vi "Main.vi"(11 "Module Admin":refnum<class "Delacor_lib_QMH_Module Admin.lvclass">) -> ()   [LabVIEW 2018, in "DMM Module.lvlib"]
doc: "This template is based off of the Queued Message Handler design pattern and the Queued Message Handler project template that ships with LabVIEW.\n\nThe main difference is that the queue is private to this module and communication between modules is performed via Broadcast and Request events.\n\nRequest events are wrapped in public API methods and are handled in the Event Handling Loop (EHL) of this VI. Any module can register for Broadcast events sent by this module. The EHL generates messages based on user interface actions.\n\nThe Message Handling Loop (MHL) processes messages generated by the EHL, or by other messages. The messages are string values, so new messages can be added easily to the Message Cases case structure in the MHL. Each message cluster can also provide an optional value for Message Data, which is a variant that can be converted to whatever message-specific data is required.\n_____\nBased on DQMH Project Template 6.0.0.91."
uses:
  DMM Module.lvlib
  <vilib>/Delacor/Delacor QMH/Libraries/Module Admin_class/Delacor_lib_QMH_Module Admin.lvclass
  Module Data--cluster.ctl
  <vilib>/Delacor/Delacor QMH/Libraries/Message Queue_class/Delacor_lib_QMH_Message Queue.lvclass/Delacor_lib_QMH_Message Queue.ctl
  Stop Argument--cluster.ctl
  <vilib>/Delacor/Delacor QMH/Libraries/Module Admin_class/Delacor_lib_QMH_Module Admin.lvclass/Delacor_lib_QMH_Module Admin.ctl
  DMM init Argument--cluster.ctl
  config channel Argument--cluster.ctl
  Read DCV_DCI Argument--cluster.ctl
  Read DCV_DCI (Reply Payload)--cluster.ctl
  DMM Close Argument--cluster.ctl
  <vilib>/Utility/miscctls.llb/LVPointTypeDef.ctl
  <vilib>/Delacor/Delacor QMH/Libraries/Message Queue_class/Delacor_lib_QMH_Enqueue Message (Single).vi
  <vilib>/Delacor/Delacor QMH/Libraries/Module Admin_class/Delacor_lib_QMH_Get External Launch.vi
  <vilib>/Utility/error.llb/Error Cluster From Error Code.vi
  <vilib>/ErrorRing/Error Ring.xnode
  <vilib>/Delacor/Delacor QMH/Libraries/Message Queue_class/Delacor_lib_QMH_Message Queue.lvclass
  <instrlib>/DMM4/DMM4.lvlib
panel:
  in  "Sets to Display":u16(ring)=2 items=["1st Display", "2nd Display", "1st & 2nd Display"]
  out "DCI":dbl
  out "DCV":dbl
  in  "Read DCV, DCI Dual mode":bool
  in  "Config Channel":bool
  in  "Detector Rate":u8(ring) items=["SLOW", "MID", "FAST"]
  in  "DCI Range":dbl=0.5
  in  "DCV Range":dbl=200.0
  in  "Open&Init":bool caption="Open&init"
  in  "VISA resource name":refnum<visa-resource-name>
  out "error out":errorcluster
  out "Status":string
  in  "Simulate MHL Error":bool
  in  "Simulate EHL Error":bool
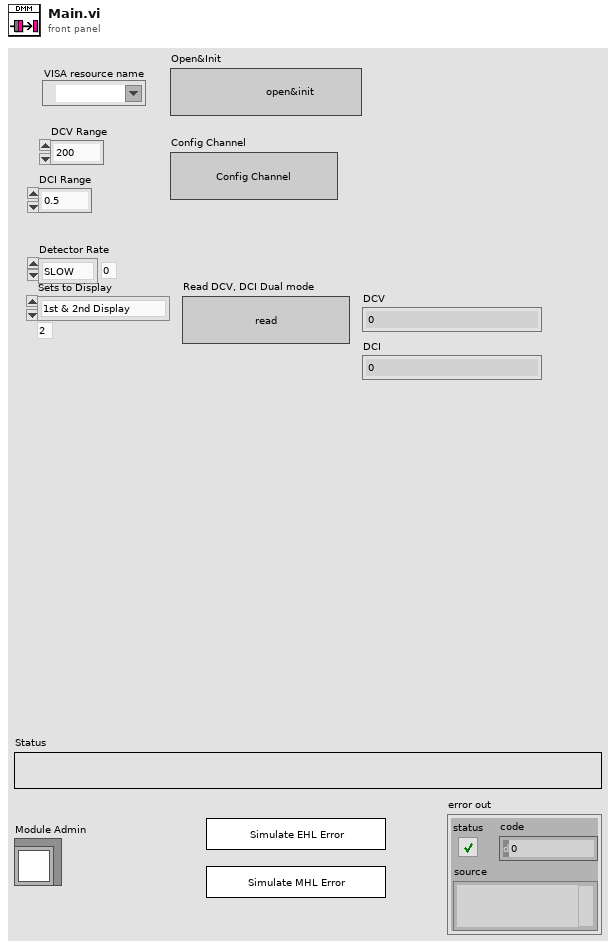
[diagram p1: front panel]
types:
  T1 = typedef "DMM Module.lvlib/Request Events--cluster.ctl" = cluster{"Stop Module":refnum<user-event>, "Do Something Else":refnum<user-event>, "Do Something Else and Wait for Reply":refnum<user-event>, "Show Panel":refnum<user-event>, "Hide Panel":refnum<user-event>, "Get Module Execution Status":refnum<user-event>, "Show Diagram":refnum<user-event>, "DMM init":refnum<user-event>, "config channel":refnum<user-event>, "Read DCV_DCI":refnum<user-event>, "DMM Close":refnum<user-event>}
  T2 = typedef "DMM Module.lvlib/Module Data--cluster.ctl" = cluster{"Status":string, "DMM  name":refnum<visa-resource-name>}
  T3 = typedef "LVPointTypeDef.ctl" = cluster{"Horizontal":i16, "Vertical":i16}
  T4 = enum32{"Invalid", "Standard", "Closed", "Hidden", "Minimized", "Maximized"}
  T5 = typedef "DMM Module.lvlib/DMM init Argument--cluster.ctl" = cluster{"VISA resource name":refnum<visa-resource-name>}
  T6 = typedef "DMM Module.lvlib/config channel Argument--cluster.ctl" = cluster{"Boolean":bool, "DCV range":dbl, "DCI range ":dbl, "Detector Rate":u8}
  T7 = typedef "DMM Module.lvlib/Read DCV_DCI (Reply Payload)--cluster.ctl" = cluster{"DCV":dbl, "DCI":dbl, "Read DCV_DCI_error":errorcluster}
  T8 = typedef "DMM Module.lvlib/Read DCV_DCI Argument--cluster.ctl" = cluster{"Wait Notifier":refnum<notifier>, "wait for reply":bool, "Sets to Display":u16}
  T9 = typedef "DMM Module.lvlib/DMM Close Argument--cluster.ctl" = cluster{"Boolean":bool}
  T10 = typedef "DMM Module.lvlib/Stop Argument--cluster.ctl" = cluster{"Origin":string, "Exit via Stop Module Req?":bool, "Wait for Module to stop?":bool}
  T11 = enum32{"invalid lock state", "Not Locked", "Locked (No Password)", "Password-protected"}
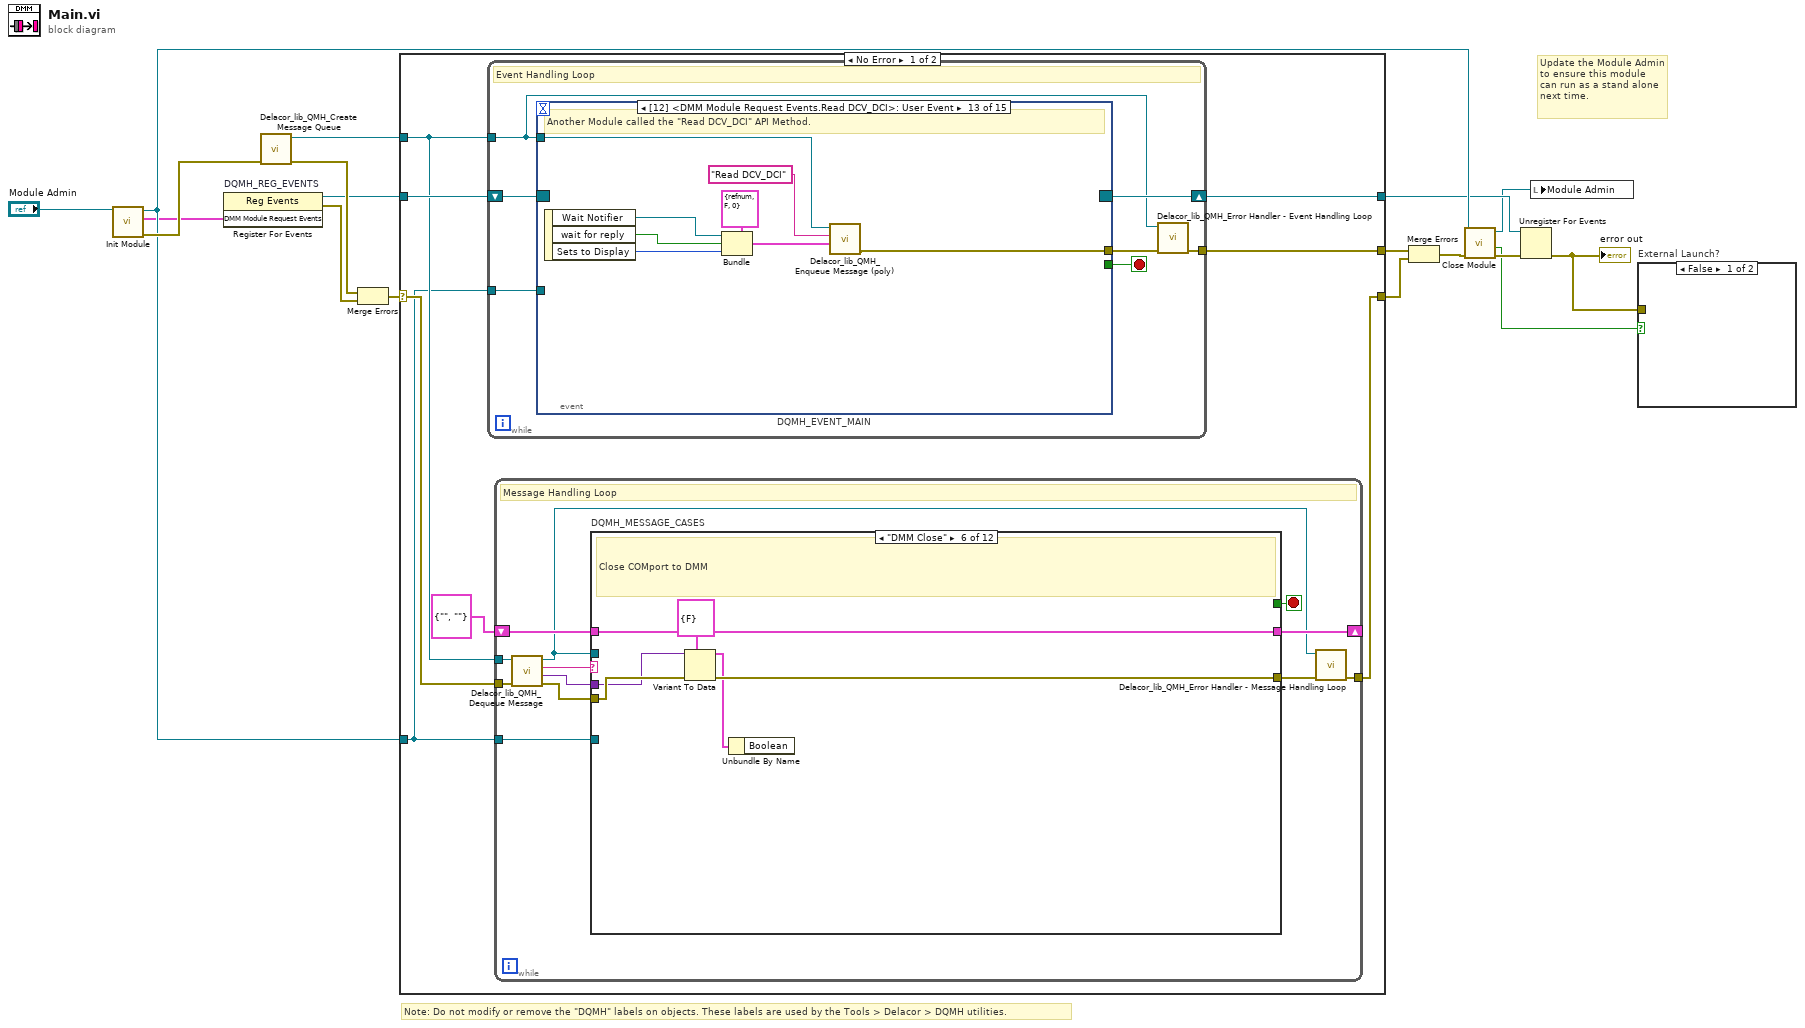
[diagram p0: block diagram]
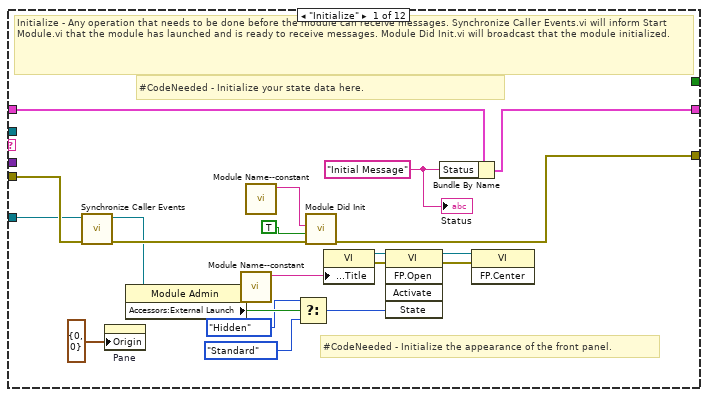
[diagram p2: hidden frame]
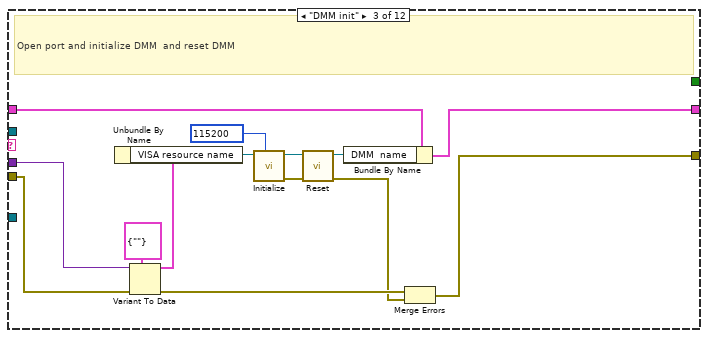
[diagram p4: hidden frame]
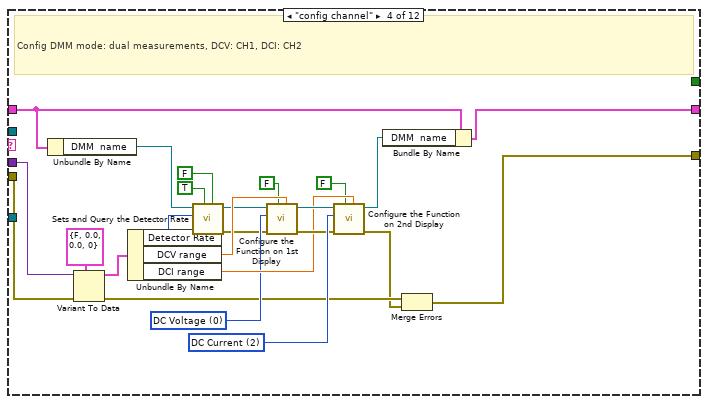
[diagram p5: hidden frame]
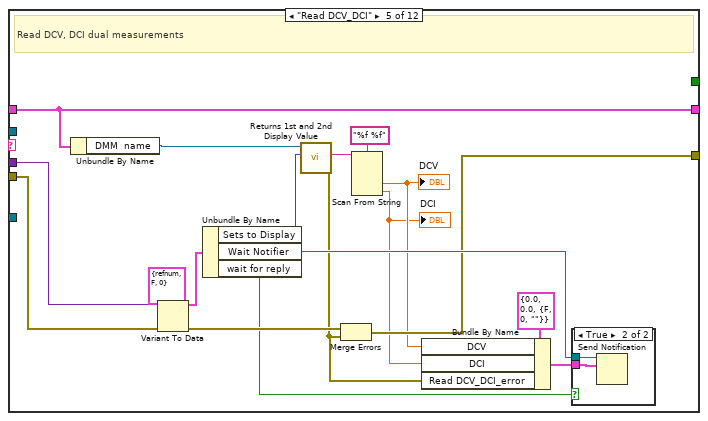
[diagram p6: hidden frame]
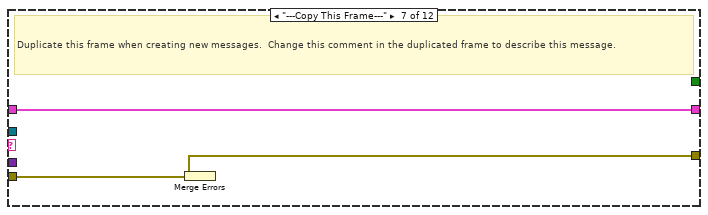
[diagram p8: hidden frame]
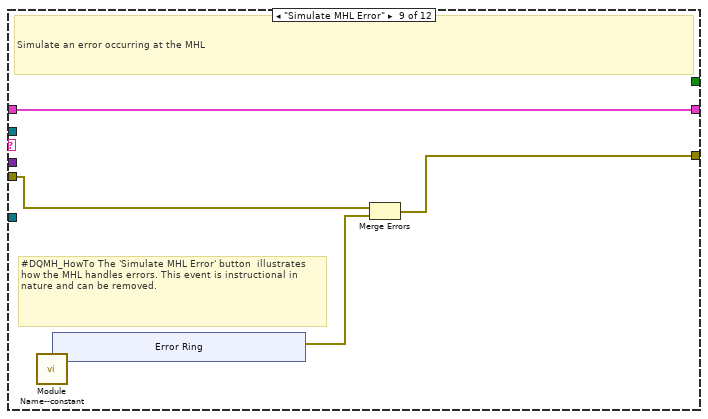
[diagram p10: hidden frame]
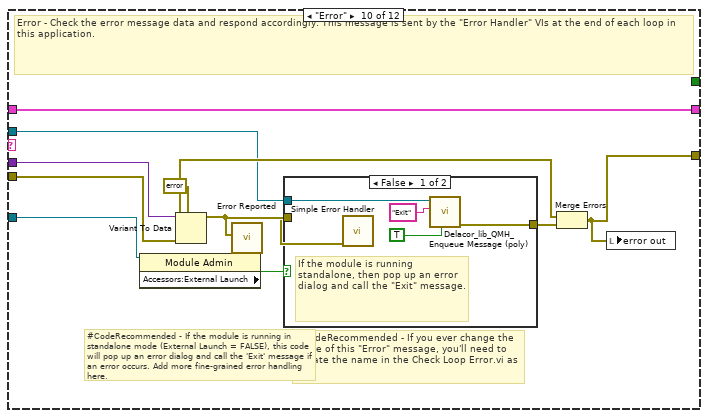
[diagram p11: hidden frame]
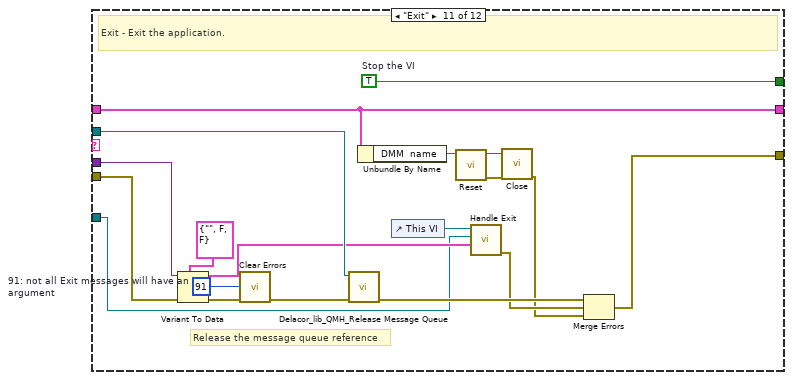
[diagram p13: hidden frame]
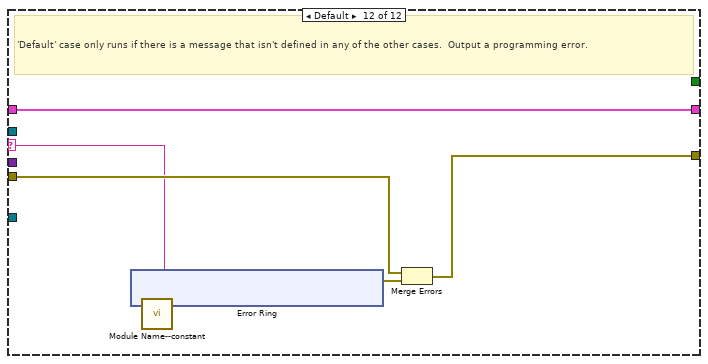
[diagram p14: hidden frame]
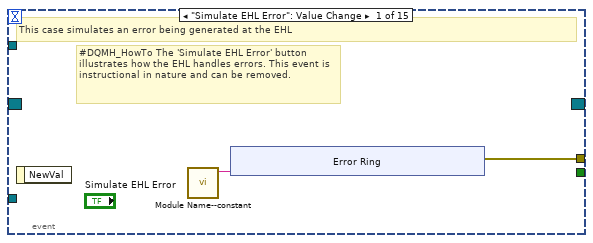
[diagram p15: hidden frame]
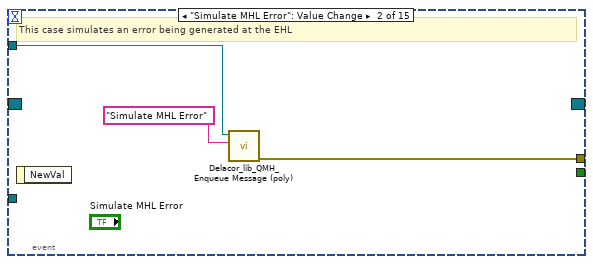
[diagram p16: hidden frame]
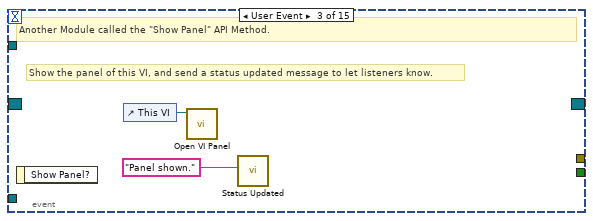
[diagram p17: hidden frame]
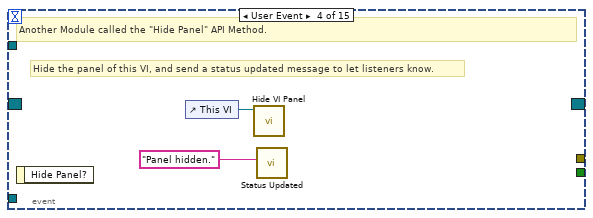
[diagram p18: hidden frame]
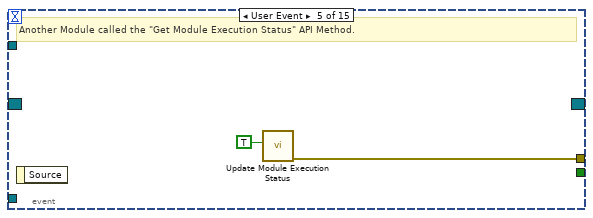
[diagram p19: hidden frame]
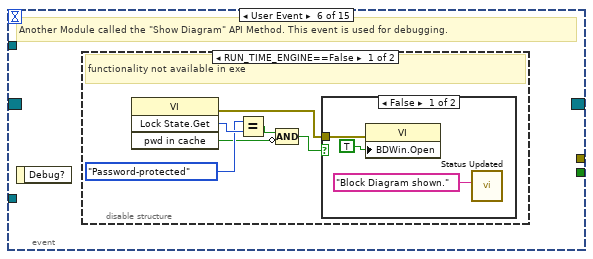
[diagram p20: hidden frame]
diagram:
  # "Note: Do not modify or remove the \"DQMH\" labels on objects. These labels are used by the Tools > Delacor > DQMH utilities."
  # "Update the Module Admin to ensure this module can run as a stand alone next time."
  n1 = call "Init Module.vi"("Singleton Module Admin in"="Module Admin") -> ("error out"=w16:errorcluster, "DMM Module Request Events"=w5:T1, "Singleton Module Admin out"=w8:refnum<class "Delacor_lib_QMH_Module Admin.lvclass">)  [unwired: 8 in]
  n2 = register-events "DQMH_REG_EVENTS"(w5) -> (reference out=w6:refnum<event-registration>, error out=w9:errorcluster)  [unwired: 2 in]
  n3 = call <vilib>:"Delacor_lib_QMH_Create Message Queue.vi"("error in"=w16) -> ("error out"=w11:errorcluster, "Message Queue"=w4:refnum<class "Delacor_lib_QMH_Message Queue.lvclass">)  [unwired: 9 in]
  n4 = Merge Errors(w11, w9) -> (w10:errorcluster)
  n5 = case shown="No Error" w10 {
    selector: w10 -> [w23 w297]
    tunnel: [w25 w296] -> w17
    tunnel: [w22 w302] -> w7
    tunnel: w6 -> [w20 w302]
    tunnel: w4 -> [w19 w295]
    tunnel: [w24 _] -> w14
    tunnel: w8 -> [w18 w298]
    frame No Error {
      n6 = while {
        tunnel: w19 -> [w190]
        shift-right: [w193] -> w22
        shift-left: w20 -> [w194]
        tunnel: [w195] -> w24
        tunnel: w18 -> [w191]
        stop <- w192 stop-if-true
        # "Event Handling Loop"
        n7 = event "DQMH_EVENT_MAIN" shown="[12] <DMM Module Request Events.Read DCV_DCI>: User Event" {
          selector: w194 -> [_ _ _ _ _ _ _ _ _ _ _ _ _ _ _]
          dyn-events: [_ _ _ _ _ _ _ _ _ _ _ _ _ _ _] -> w193
          timeout: _ -> [_ _ _ _ _ _ _ _ _ _ _ _ _ _ _]
          tunnel: [_ _ _ _ _ _ TRUE ("Discard?") _ _ _ _ _ _ _ _] -> w192
          tunnel: w190 -> [_ w207 _ _ _ _ w224 w238 w251 w256 w266 w269 w282 w288 w294]
          tunnel: [w198 w208 _ _ w214 _ w234 w240 w246 w252 w261 w267 w276 w283 w289] -> w196
          tunnel: w191 -> [_ _ _ _ _ _ _ w237 _ _ _ _ _ _ _]
          event "Simulate EHL Error": Value Change {
            # "#DQMH_HowTo The 'Simulate EHL Error' button  illustrates how the EHL handles errors. This event is instructional in nature and can be removed."
            # "This case simulates an error being generated at the EHL"
            n8 = event-data() -> ()  [unwired: 1 in, 1 out]
            n9 = call "Module Name--constant.vi"() -> ("Module Name"=w197:string)  [unwired: 11 in]
            n10 = xnode "Error Ring"("parameter 0"=w197) -> ("error out"=w198:errorcluster)
          }
          event "Simulate MHL Error": Value Change {
            # "This case simulates an error being generated at the EHL"
            n11 = event-data() -> ()  [unwired: 1 in, 1 out]
            n12 = call-poly <vilib>:"Delacor_lib_QMH_Enqueue Message (poly).vi"("Message"="Simulate MHL Error", "Message Queue in"=w207) -> ("error out"=w208:errorcluster)  [unwired: 8 in, 1 out]
          }
          event User Event {
            # "Show the panel of this VI, and send a status updated message to let listeners know."
            # "Another Module called the \"Show Panel\" API Method."
            n13 = event-data() -> ()  [unwired: 1 in, 1 out]
            n14 = control-ref of="This VI"() -> (w210:refnum<vi>)
            n15 = call "Open VI Panel.vi"("VI"=w210) -> ()  [unwired: 10 in, 1 out]
            n16 = call "Status Updated.vi"("Status"="Panel shown." ("format string")) -> ()  [unwired: 10 in, 1 out]
          }
          event User Event {
            # "Hide the panel of this VI, and send a status updated message to let listeners know."
            # "Another Module called the \"Hide Panel\" API Method."
            n17 = event-data() -> ()  [unwired: 1 in, 1 out]
            n18 = control-ref of="This VI"() -> (w212:refnum<vi>)
            n19 = call "Hide VI Panel.vi"("VI"=w212) -> ()  [unwired: 10 in, 1 out]
            n20 = call "Status Updated.vi"("Status"="Panel hidden." ("format string")) -> ()  [unwired: 10 in, 1 out]
          }
          event User Event {
            # "Another Module called the \"Get Module Execution Status\" API Method."
            n21 = event-data() -> ()  [unwired: 1 in, 1 out]
            n22 = call "Update Module Execution Status.vi"("Running?"=TRUE) -> ("error out"=w214:errorcluster)  [unwired: 10 in]
          }
          event User Event {
            # "Another Module called the \"Show Diagram\" API Method. This event is used for debugging."
            n23 = event-data() -> ()  [unwired: 1 in, 1 out]
            n24 = disable-structure shown="RUN_TIME_ENGINE==False" {
              frame condition #0 (active) {
                # "functionality not available in exe"
                n25 = invoke class="VI" method="Lock State.Get"() -> (error out=w220:errorcluster, "Get Lock State"=w219:T11, "pwd in cache"=w216:bool)  [unwired: 4 in, 1 out]
                n26 = Equal?(x=T11."Password-protected", y=w219) -> (x = y?=w217:bool)
                n27 = Compound Arithmetic op=AND(w217, invert w216) -> (w215:bool)
                n28 = case shown="False" w215 {
                  tunnel: w220 -> [w223 _]
                  frame False {
                    n29 = property class="VI"(error in=w223, "BDWin.Open"=TRUE ("Block Diagram Window:Open")) -> ()  [unwired: 1 in, 2 out]
                    n30 = call "Status Updated.vi"("Status"="Block Diagram shown." ("format string")) -> ()  [unwired: 10 in, 1 out]
                  }
                  frame True {
                    # "Password-protected VI, and the password is not in the cache. Do not show the diagram."
                  }
                }
              }
              frame condition #1 {
              }
            }
          }
          event User Event {
            # "The Stop Module Event can get fired from the Exit message in the MHL. The queue gets destroyed in that case. If the queue no longer exists, the Enqueue Exit as a priority message will return error 1. It is safe to ignore, because the module is already exiting."
            # "Another Module called the \"Stop Module\" API Method  or the Message Handling Loop below."
            n31 = event-data() -> ("Origin"=w231:string, "Exit via Stop Module Req?"=w227:bool, "Wait for Module to stop?"=w226:bool)  [unwired: 1 in]
            n32 = local write "Status"(w231) -> ()
            n33 = Bundle By Name(cluster=T10 {"Origin"="", "Exit via Stop Module Req?"=FALSE, "Wait for Module to stop?"=FALSE} ("Stop Argument"), "Exit via Stop Module Req?"=w227, "Wait for Module to stop?"=w226) -> (w225:T10)
            n34 = call-poly <vilib>:"Delacor_lib_QMH_Enqueue Message (poly).vi"("Priority Message? (F)"=TRUE, "Message Data"=w225, "Message"="Exit", "Message Queue in"=w224) -> ("error out"=w235:errorcluster)  [unwired: 6 in, 1 out]
            n35 = call <vilib>:"Clear Errors.vi"("error in (no error)"=w235, "specific error code to clear (0: all)"=1) -> ("error out"=w234:errorcluster)  [unwired: 4 in, 1 out]
          }
          event Panel Close? {
            w239 = TRUE  # Discard the event, the MHL is responsible for closing and stopping this VI.
            # "Hide the panel or send the 'Exit' message if the user clicks the 'X' on the module main VI panel."
            n36 = event-data() -> ()  [unwired: 1 in, 1 out]
            n37 = property class="Module Admin"(reference=w237) -> ("Accessors:External Launch"=w236:bool)  [unwired: 1 in, 2 out]
            n38 = case shown="False" w236 {
              tunnel: w238 -> [_ w244]
              tunnel: [_ w245] -> w240
              frame True {
                # "If externally launched, clicking the 'X' hides the panel, but doesn't close it."
                n39 = control-ref of="This VI"() -> (w241:refnum<vi>)
                n40 = call "Hide VI Panel.vi"("VI"=w241) -> ()  [unwired: 10 in, 1 out]
              }
              frame False {
                # "If run as a stand-alone VI, clicking the panel 'X' stops the VI."
                n41 = call-poly <vilib>:"Delacor_lib_QMH_Enqueue Message (poly).vi"("Priority Message? (F)"=TRUE, "Message"="Exit", "Message Queue in"=w244) -> ("error out"=w245:errorcluster)  [unwired: 7 in, 1 out]
              }
            }
            n42 = event-data("Discard?"=w239) -> ()  [unwired: 1 in, 1 out]
          }
          event User Event {
            # "Another Module called the \"DMM init\" API Method."
            n43 = event-data() -> ("VISA resource name"=w247:refnum<visa-resource-name>)  [unwired: 1 in]
            n44 = Bundle(cluster=T5 {"VISA resource name"=""} ("DMM init Argument"), "VISA resource name"=w247) -> (w248:T5)
            n45 = call-poly <vilib>:"Delacor_lib_QMH_Enqueue Message (poly).vi"("Message Data"=w248, "Message"="DMM init", "Message Queue in"=w251) -> ("error out"=w246:errorcluster)  [unwired: 7 in, 1 out]
          }
          event "Open&Init": Value Change {
            n46 = event-data() -> ()  [unwired: 1 in, 1 out]
            n47 = Bundle By Name(cluster=T5 {"VISA resource name"=""} ("DMM init Argument"), "VISA resource name"="VISA resource name") -> (w253:T5)
            n48 = call-poly <vilib>:"Delacor_lib_QMH_Enqueue Message (poly).vi"("Message Data"=w253, "Message"="DMM init", "Message Queue in"=w256) -> ("error out"=w252:errorcluster)  [unwired: 7 in, 1 out]
          }
          event User Event {
            # "Another Module called the \"config channel\" API Method."
            n49 = event-data() -> ("Boolean"=w262:bool, "DCV range"=w260:dbl, "DCI range"=w259:dbl, "Detector Rate"=w258:u8)  [unwired: 1 in]
            n50 = Bundle(cluster=T6 {"Boolean"=FALSE, "DCV range"=0.0, "DCI range "=0.0, "Detector Rate"=0} ("config channel Argument"), "Boolean"=w262, "DCV range"=w260, "DCI range"=w259, "Detector Rate"=w258) -> (w263:T6)
            n51 = call-poly <vilib>:"Delacor_lib_QMH_Enqueue Message (poly).vi"("Message Data"=w263, "Message"="config channel", "Message Queue in"=w266) -> ("error out"=w261:errorcluster)  [unwired: 7 in, 1 out]
          }
          event "Config Channel": Value Change {
            n52 = event-data() -> ()  [unwired: 1 in, 1 out]
            n53 = Bundle By Name(cluster=T6 {"Boolean"=FALSE, "DCV range"=0.0, "DCI range "=0.0, "Detector Rate"=0} ("config channel Argument"), "DCV range"="DCV Range", "DCI range"="DCI Range", "Detector Rate"="Detector Rate") -> (w268:T6)
            n54 = call-poly <vilib>:"Delacor_lib_QMH_Enqueue Message (poly).vi"("Message Data"=w268, "Message"="config channel", "Message Queue in"=w269) -> ("error out"=w267:errorcluster)  [unwired: 7 in, 1 out]
          }
          event User Event {
            # "Another Module called the \"Read DCV_DCI\" API Method."
            n55 = event-data() -> ("Wait Notifier"=w278:refnum<notifier>, "wait for reply"=w277:bool, "Sets to Display"=w275:u16)  [unwired: 1 in]
            n56 = Bundle(cluster=T8 {"Wait Notifier"=refnum, "wait for reply"=FALSE, "Sets to Display"=0} ("Read DCV_DCI Argument"), "Wait Notifier"=w278, "wait for reply"=w277, "Sets to Display"=w275) -> (w279:T8)
            n57 = call-poly <vilib>:"Delacor_lib_QMH_Enqueue Message (poly).vi"("Message Data"=w279, "Message"="Read DCV_DCI", "Message Queue in"=w282) -> ("error out"=w276:errorcluster)  [unwired: 7 in, 1 out]
          }
          event "Read DCV, DCI Dual mode": Value Change {
            n58 = event-data() -> ()  [unwired: 1 in, 1 out]
            n59 = Bundle By Name(cluster=T8 {"Wait Notifier"=refnum, "wait for reply"=FALSE, "Sets to Display"=0} ("Read DCV_DCI Argument"), "Sets to Display"="Sets to Display") -> (w284:T8)
            n60 = call-poly <vilib>:"Delacor_lib_QMH_Enqueue Message (poly).vi"("Message Data"=w284, "Message"="Read DCV_DCI", "Message Queue in"=w288) -> ("error out"=w283:errorcluster)  [unwired: 7 in, 1 out]
          }
          event User Event {
            # "Another Module called the \"DMM Close\" API Method."
            n61 = event-data() -> ("Boolean"=w290:bool)  [unwired: 1 in]
            n62 = Bundle(cluster=T9 {"Boolean"=FALSE} ("DMM Close Argument"), "Boolean"=w290) -> (w291:T9)
            n63 = call-poly <vilib>:"Delacor_lib_QMH_Enqueue Message (poly).vi"("Message Data"=w291, "Message"="DMM Close", "Message Queue in"=w294) -> ("error out"=w289:errorcluster)  [unwired: 7 in, 1 out]
          }
        }
        n64 = call-dynamic "Delacor_lib_QMH_Error Handler - Event Handling Loop.vi"("error in"=w196, "Message Queue in"=w190) -> ("dup error in"=w195:errorcluster)  [unwired: 8 in, 1 out]
      }
      n65 = while {
        tunnel: w19 -> [w28]
        shift-right: [w32] -> _
        shift-left: T2 {"Status"="", "DMM  name"=""} ("Data Cluster") -> [w33]
        tunnel: w23 -> [w36]
        tunnel: [w34] -> w25
        tunnel: w18 -> [w26]
        stop <- w31 stop-if-true
        # "Message Handling Loop"
        n66 = call-dynamic "Delacor_lib_QMH_Dequeue Message.vi"("error in"=w36, "Message Queue in"=w28) -> ("error out"=w35:errorcluster, "Message Data"=w29:variant, "Message"=w30:string, "Message Queue out"=w27:refnum<class "Delacor_lib_QMH_Message Queue.lvclass">)  [unwired: 6 in]
        n67 = case "DQMH_MESSAGE_CASES" shown="\"DMM Close\"" w30 {
          selector: w30 -> [_ _ _ _ _ _ _ _ _ _ _ w177]
          tunnel: w27 -> [_ _ _ _ _ _ _ _ _ w144 w169 _]
          tunnel: w35 -> [w55 w59 w73 w97 w115 w123 w126 w128 w133 w150 w175 w179]
          tunnel: [w53 w59 w62 w88 w106 w121 w125 w128 w132 w147 w172 w180] -> w37
          tunnel: w33 -> [w44 w58 w66 w89 w105 w122 w124 w127 w130 w146 w161 w178]
          tunnel: [w43 w58 w67 w90 w105 w122 w124 w127 w130 w146 w161 w178] -> w32
          tunnel: [_ _ _ _ _ _ _ _ _ _ w168 _] -> w31
          tunnel: w29 -> [_ _ w72 w96 w113 w120 _ _ _ w145 w167 _]
          tunnel: w26 -> [w45 _ _ _ _ _ _ _ _ w143 w162 _]
          frame "Initialize" {
            w39 = "Initial Message" ("Initial Message")
            # "#CodeNeeded - Initialize the appearance of the front panel."
            # "#CodeNeeded - Initialize your state data here."
            # "Initialize - Any operation that needs to be done before the module can receive messages. Synchronize Caller Events.vi will inform Start Module.vi that the module has launched and is ready to receive messages. Module Did Init.vi will broadcast that the module initialized."
            n68 = call "Synchronize Caller Events.vi"("error in (no error)"=w55, "Singleton Module Admin in"=w45) -> ("error out"=w54:errorcluster, "Singleton Module Admin out"=w40:refnum<class "Delacor_lib_QMH_Module Admin.lvclass">)  [unwired: 8 in]
            n69 = property on="Pane" class="Pane"("Origin"=T3 {"Horizontal"=0, "Vertical"=0}) -> ()  [unwired: 2 in, 2 out]
            n70 = property class="Module Admin"(reference=w40) -> ("Accessors:External Launch"=w49:bool)  [unwired: 1 in, 2 out]
            n71 = call "Module Name--constant.vi"() -> ("Module Name"=w52:string)  [unwired: 11 in]
            n72 = call "Module Name--constant.vi"() -> ("Module Name"=w41:string)  [unwired: 11 in]
            n73 = Select(t=T4."Hidden" ("State"), s=w49, f=T4."Standard" ("State")) -> (s? t:f=w46:T4)
            n74 = call "Module Did Init.vi"("error in (no error)"=w54, "Initialized?"=TRUE, "Origin"=w41) -> ("error out"=w53:errorcluster)  [unwired: 8 in]
            n75 = property class="VI"("Front Panel.Title"=w52) -> (reference out=w51:refnum<vi>, error out=w57:errorcluster)  [unwired: 2 in]
            n76 = invoke class="VI" method="FP.Open"(reference=w51, error in=w57, "State"=w46) -> (reference out=w50:refnum<vi>, error out=w56:errorcluster)  [unwired: 2 in, 3 out]
            n77 = Bundle By Name(cluster=w44, "Status"=w39) -> (w43:T2)
            n78 = invoke class="VI" method="FP.Center"(reference=w50, error in=w56) -> ()  [unwired: 1 in, 3 out]
            "Status" <- w39
          }
          frame "---Module Specific---" {
            # "Separator -- The following cases handle messages specific to this Module."
          }
          frame "DMM init" {
            w68 = u32 115200 items=["9600"=9600, "19200"=19200, "38400"=38400, "57600"=57600, "115200"=115200] ("Configure RS232 Baud Rate")
            # "Open port and initialize DMM  and reset DMM"
            n79 = Variant To Data(error in=w73, type=T5 {"VISA resource name"=""} ("DMM init Argument"), Variant=w72) -> (data=w70:T5, error out=w61:errorcluster)
            n80 = Unbundle By Name(w70) -> ("VISA resource name"=w69:refnum<visa-resource-name>)
            n81 = call <instrlib>:"Initialize.vi"("Configure RS232 Baud Rate"=w68, "VISA resource name"=w69) -> ("error out"=w63:errorcluster, "VISA resource name out"=w65:refnum<visa-resource-name>)  [unwired: 6 in, 2 out]
            n82 = call <instrlib>:"Reset.vi"("error in (no error)"=w63, "VISA resource name"=w65) -> ("error out"=w60:errorcluster, "VISA resource name out"=w64:refnum<visa-resource-name>)  [unwired: 8 in]
            n83 = Bundle By Name(cluster=w66, "DMM  name"=w64) -> (w67:T2)
            n84 = Merge Errors(w61, w60) -> (w62:errorcluster)
          }
          frame "config channel" {
            w92 = u8 2 items=["DC Voltage", "AC Voltage", "DC Current", "AC Current", "2-Wire Resistance", "Frequency", "Period", "None"] ("Function")
            w80 = u8 0 items=["DC Voltage", "AC Voltage", "DC+AC Voltage", "DC Current", "AC Current", "DC+AC Current", "2-Wire Resistance", "Frequency", "Period", "Continuity", "Diode", "Temperature", "Capacitance"] ("Function")
            # "Config DMM mode: dual measurements, DCV: CH1, DCI: CH2"
            n85 = Unbundle By Name(w89) -> ("DMM  name"=w85:refnum<visa-resource-name>)
            n86 = Variant To Data(error in=w97, type=T6 {"Boolean"=FALSE, "DCV range"=0.0, "DCI range "=0.0, "Detector Rate"=0} ("config channel Argument"), Variant=w96) -> (data=w94:T6, error out=w76:errorcluster)
            n87 = Unbundle By Name(w94) -> ("Detector Rate"=w84:u8, "DCV range"=w87:dbl, "DCI range"=w86:dbl)
            n88 = call <instrlib>:"Sets and Query the Detector Rate.vi"("Enable to Query"=FALSE, "Enable to Sets"=TRUE, "Detector Rate"=w84, "VISA resource name"=w85) -> ("error out"=w78:errorcluster, "VISA resource name out"=w81:refnum<visa-resource-name>)  [unwired: 5 in, 1 out]
            n89 = call <instrlib>:"Configure the Function on 1st Display .vi"("Manual Range"=w87, "Enable Auto Range"=FALSE, "error in"=w78, "Function"=w80, "VISA resource name"=w81) -> ("error out"=w91:errorcluster, "VISA resource name out"=w93:refnum<visa-resource-name>)  [unwired: 5 in]
            n90 = call <instrlib>:"Configure the Function on 2nd Display.vi"("Manual Range"=w86, "Enable Auto Range"=FALSE, "error in"=w91, "Function"=w92, "VISA resource name"=w93) -> ("error out"=w75:errorcluster, "VISA resource name out"=w74:refnum<visa-resource-name>)  [unwired: 5 in]
            n91 = Bundle By Name(cluster=w89, "DMM  name"=w74) -> (w90:T2)
            n92 = Merge Errors(w76, w75) -> (w88:errorcluster)
          }
          frame "Read DCV_DCI" {
            # "Read DCV, DCI dual measurements"
            n93 = Unbundle By Name(w105) -> ("DMM  name"=w104:refnum<visa-resource-name>)
            n94 = Variant To Data(error in=w115, type=T8 {"Wait Notifier"=refnum, "wait for reply"=FALSE, "Sets to Display"=0} ("Read DCV_DCI Argument"), Variant=w113) -> (data=w111:T8, error out=w114:errorcluster)
            n95 = Unbundle By Name(w111) -> ("Sets to Display"=w103:u16, "Wait Notifier"=w110:refnum<notifier>, "wait for reply"=w109:bool)
            n96 = call <instrlib>:"Returns 1st and 2nd Display Value.vi"("Sets to Display"=w103, "VISA resource name"=w104) -> ("error out"=w100:errorcluster, "Return the Value"=w101:string)  [unwired: 7 in, 1 out]
            n97 = Merge Errors(w114, w100) -> (w106:errorcluster)
            n98 = Scan From String(format string="%f %f", input string=w101) -> (output 1=w99:dbl, output 2=w98:dbl)  [unwired: 4 in, 3 out]
            "DCV" <- w99
            "DCI" <- w98
            n99 = Bundle By Name(cluster=T7 {"DCV"=0.0, "DCI"=0.0, "Read DCV_DCI_error"={"status"=FALSE, "code"=0, "source"=""}} ("Read DCV_DCI (Reply Payload)"), "DCV"=w99, "DCI"=w98, "Read DCV_DCI_error"=w100) -> (w108:T7)
            n100 = case shown="True" w109 {
              tunnel: w110 -> [_ w117]
              tunnel: w108 -> [_ w116]
              frame False {
              }
              frame True {
                n101 = Send Notification(notification=w116, notifier=w117) -> ()  [unwired: 1 in, 2 out]
              }
            }
          }
          frame "DMM Close" {
            # "Close COMport to DMM"
            n102 = Variant To Data(error in=w123, type=T9 {"Boolean"=FALSE} ("DMM Close Argument"), Variant=w120) -> (data=w118:T9, error out=w121:errorcluster)
            n103 = Unbundle By Name(w118) -> ()  [unwired: 1 out]
          }
          frame "---Copy This Frame---" {
            # "Duplicate this frame when creating new messages.  Change this comment in the duplicated frame to describe this message."
            n104 = Merge Errors(w126) -> (w125:errorcluster)
          }
          frame "---Exit and Error Handling---" {
            # "Separator - The following cases handle errors and exit messages."
          }
          frame "Simulate MHL Error" {
            # "#DQMH_HowTo The 'Simulate MHL Error' button  illustrates how the MHL handles errors. This event is instructional in nature and can be removed."
            # "Simulate an error occurring at the MHL"
            n105 = call "Module Name--constant.vi"() -> ("Module Name"=w129:string)  [unwired: 11 in]
            n106 = xnode "Error Ring"("parameter 0"=w129) -> ("error out"=w131:errorcluster)
            n107 = Merge Errors(w133, w131) -> (w132:errorcluster)
          }
          frame "Error" {
            # "#CodeRecommended - If you ever change the name of this \"Error\" message, you'll need to update the name in the Check Loop Error.vi as well."
            # "#CodeRecommended - If the module is running in standalone mode (External Launch = FALSE), this code will pop up an error dialog and call the 'Exit' message if an error occurs. Add more fine-grained error handling here."
            # "Error - Check the error message data and respond accordingly. This message is sent by the \"Error Handler\" VIs at the end of each loop in this application."
            n108 = property class="Module Admin"(reference=w143) -> ("Accessors:External Launch"=w142:bool)  [unwired: 1 in, 2 out]
            n109 = Variant To Data(error in=w150, type=errorcluster {"status"=FALSE, "code"=0, "source"=""} ("error constant"), Variant=w145) -> (data=w151:errorcluster, error out=w148:errorcluster)
            n110 = call "Error Reported.vi"("Error"=w151) -> ()  [unwired: 10 in, 1 out]
            n111 = case shown="False" w142 {
              tunnel: [w156 _] -> w141
              tunnel: w144 -> [w154 _]
              tunnel: w151 -> [w155 _]
              frame False {
                # "If the module is running standalone, then pop up an error dialog and call the \"Exit\" message."
                n112 = call <vilib>:"Simple Error Handler.vi"("error in (no error)"=w155) -> ()  [unwired: 4 in, 5 out]
                n113 = call-poly <vilib>:"Delacor_lib_QMH_Enqueue Message (poly).vi"("Priority Message? (F)"=TRUE, "Message"="Exit", "Message Queue in"=w154) -> ("error out"=w156:errorcluster)  [unwired: 7 in, 1 out]
              }
              frame True {
                # "If the module was launched externally, calling the Error Reported broadcast VI is the only action performed by the \"Error\" message. The module's caller can then process the error appropriately."
              }
            }
            n114 = Merge Errors(w148, w141) -> (w147:errorcluster)
            n115 = local write "error out"(w147) -> ()
          }
          frame "Exit" {
            w166 = 91  # 91: not all Exit messages will have an argument
            w168 = TRUE  # Stop the VI
            # "Release the message queue reference"
            # "Exit - Exit the application."
            n116 = Variant To Data(error in=w175, type=T10 {"Origin"="", "Exit via Stop Module Req?"=FALSE, "Wait for Module to stop?"=FALSE} ("Stop Argument"), Variant=w167) -> (data=w164:T10, error out=w171:errorcluster)
            n117 = call <vilib>:"Clear Errors.vi"("error in (no error)"=w171, "specific error code to clear (0: all)"=w166) -> ("error out"=w174:errorcluster)  [unwired: 4 in, 1 out]
            n118 = call-dynamic "Delacor_lib_QMH_Release Message Queue.vi"("error in"=w174, "Message Queue"=w169) -> ("error out"=w173:errorcluster)  [unwired: 9 in]
            n119 = Unbundle By Name(w161) -> ("DMM  name"=w159:refnum<visa-resource-name>)
            n120 = control-ref of="This VI"() -> (w163:refnum<vi>)
            n121 = call <instrlib>:"Reset.vi"("VISA resource name"=w159) -> ("error out"=w157:errorcluster, "VISA resource name out"=w158:refnum<visa-resource-name>)  [unwired: 9 in]
            n122 = call "Handle Exit.vi"("Stop Argument"=w164, "Admin in"=w162, "VI reference"=w163) -> ("error out"=w170:errorcluster)  [unwired: 7 in, 1 out]
            n123 = call <instrlib>:"Close.vi"("error in (no error)"=w157, "VISA resource name"=w158) -> ("error out"=w160:errorcluster)  [unwired: 9 in]
            n124 = Merge Errors(w173, w170, w160) -> (w172:errorcluster)
          }
          frame Default {
            # "'Default' case only runs if there is a message that isn't defined in any of the other cases.  Output a programming error."
            n125 = call "Module Name--constant.vi"() -> ("Module Name"=w176:string)  [unwired: 11 in]
            n126 = xnode "Error Ring"("parameter 0"=w177, "parameter 1"=w176) -> ("error out"=w181:errorcluster)
            n127 = Merge Errors(w179, w181) -> (w180:errorcluster)
          }
        }
        n128 = call-dynamic "Delacor_lib_QMH_Error Handler - Message Handling Loop.vi"("error in"=w37, "Message Queue in"=w27) -> ("dup error in"=w34:errorcluster)  [unwired: 8 in, 1 out]
      }
    }
    frame Error {
      # "Synchronize Caller Events.vi will inform Start Module.vi that the module has launched and will let the code calling Start Module.vi register for broadcasts and would permit the caller receive the broadcast that an error occurred at launch time."
      n129 = call "Synchronize Caller Events.vi"("Singleton Module Admin in"=w298) -> ("error out"=w303:errorcluster)  [unwired: 9 in, 1 out]
      n130 = call-dynamic "Delacor_lib_QMH_Release Message Queue.vi"("error in"=w297, "Message Queue"=w295) -> ("error out"=w296:errorcluster)  [unwired: 9 in]
      n131 = call "Module Name--constant.vi"() -> ("Module Name"=w301:string)  [unwired: 11 in]
      n132 = Merge Errors(w296, w303) -> (w304:errorcluster)
      n133 = Format Into String(format string="An error occurred during initialization. %s is no longer running.", w301) -> (resulting string=w299:string)  [unwired: 2 in, 1 out]
      n134 = call "Error Reported.vi"("Additional Information"=w299, "Error"=w304) -> ()  [unwired: 9 in, 1 out]
    }
  }
  n135 = Merge Errors(w14, w17) -> (w13:errorcluster)
  n136 = call "Close Module.vi"("error in (no error)"=w13, "Module Admin in"=w8) -> ("error out"=w15:errorcluster, "External Launch"=w1:bool, "Module Admin out"=w2:refnum<class "Delacor_lib_QMH_Module Admin.lvclass">)  [unwired: 7 in]
  n137 = Unregister For Events(event registration refnum=w7, error in=w15) -> (error out=w12:errorcluster)
  "error out" <- w12
  n138 = local write "Module Admin"(w2) -> ()
  n139 = case "External Launch?" shown="False" w1 {
    tunnel: w12 -> [_ w305]
    frame False {
    }
    frame True {
      n140 = case shown="Error" w305 {
        frame No Error {
          n141 = invoke class="VI" method="FP.Close"() -> ()  [unwired: 3 in, 3 out]
        }
        frame Error {
          n142 = invoke class="VI" method="FP.Open"("Activate"=TRUE ("Activate?")) -> ()  [unwired: 4 in, 5 out]
        }
      }
    }
  }
